vi "CompareRegenModes.vi"() -> ()   [LabVIEW 2014]
doc: "I. Description:\nThis example demonstrates how to continuously output a waveform using an internal sample clock. The automatic regeneration of data has been disabled, so new data has to be provided throughout the duration of the continuous Analog Output operation. This allows the generation of any arbitrary frequency as this VI computes new data for each iteration of the loop, maintaining phase continuity of the signal. The regeneration of data has also been adjusted so that the newest data is output as quickly as possible; thus reducing the lag between the changing of the data and the output of that data.\n\nII. Instructions for Running:\n1. Select the Physical Channel to correspond to where your signal is output on the DAQ device.\n2. Enter the Minimum and Maximum Voltage range.\n3. Specify the desired Sample Clock Rate of the output Waveform. Higher sample clock rates will produce a smoother waveform.\n4. Manually specify the Analog Output buffer size, in number of samples. A larger buffer would help non-regenerative operations avoid errors due to occasional high CPU load. \nNote: \nThe Analog Output buffer has to be at least as big as the amount of data being written to the board per iteration. The recommended buffer size would be at least twice the amount of data being written to the board per iteration.\n5. Enter the Waveform Information. See the documentation of the Basic Function Generator SubVI for information on each parameter.\n\nIII. Block Diagram Steps:\n1. Create an Analog Output Voltage channel.\n2. Configure the task to prohibit the automatic regeneration of data.\n2a. Set the transfer condition to Less than Full. Allows for more rapid updates of Output Buffer.\n3. Call the DAQmx (Sample Clock) VI to set the sample clock rate. Additionally, set the sample mode to Continuous.\n4. Read the actual sample clock rate (eventually coerced depending on the hardware used). \n5. Compute the desired waveform, using the buffer size and the actual update rate. This VI keeps track of the phase of the waveform to ensure that the generated signal is continuous.\n6. Write the waveform to the output buffer. \n7a. Call the Start VI. This is only needed when the loop is executed for the first time.\n7b. Do nothing.\n8. Loop continuously until user presses the Stop button. Every iteration computes and writes a new waveform to the buffer.\n9. Call the Clear Task VI to clear the Task.\n10. Use the popup dialog box to display an error or warning if any.\n\nIV. I/O Connections Overview:\nMake sure your signal output terminal matches the Physical Channel I/O Control. For further connection information, refer to your hardware reference manual."
uses:
  <vilib>/Utility/error.llb/DialogType.ctl
  <vilib>/DAQmx/create/channels.llb/DAQmx Create Virtual Channel.vi
  <vilib>/DAQmx/configure/timing.llb/DAQmx Timing.vi
  <vilib>/DAQmx/write.llb/DAQmx Write.vi
  <vilib>/measure/NI_MABase.lvlib
  <resource>/objmgr/daqmx.rc
panel:
  in  "Regeneration Mode":i32(ring)=10158 items=["Allow Regeneration"=10097, "Do Not Allow Regeneration"=10158]
  in  "Update Buffer":bool
  in  "Stupid Pause":bool
  in  "Size (Samples)":u32=5000
  out "Actual Sample Clock Rate":dbl=20000.0 format="%.2f"
  in  "Sample Clock Rate":dbl=20000.0 format="%0.2f"
  in  "Waveform Type":T1(ring)
  in  "Frequency":dbl=997.0 format="%.2f"
  in  "Amplitude":dbl=1.0 format="%0.2p"
  out "Waveform Graph":waveform(dbl)(graph)={"t0"=timestamp(12.75 s since 1904-01-01), "dt"=5e-05, "Y"=[]} caption="Output Waveform"
  in  "Physical Channels":tag="Dev1/ao0"
  in  "Minimum Value":dbl=-10.0 format="%0.2f"
  in  "Maximum Value":dbl=10.0 format="%0.2f"
  in  "stop":bool
  # "For instructions, select Help>>Show Context Help"
  # "Channel Parameters"
  # "Timing Parameters"
  # "Buffer Parameters"
  # "Waveform Information"
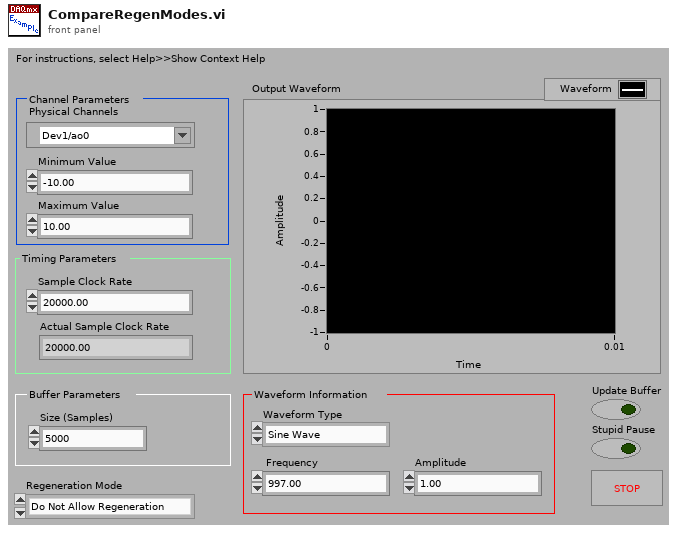
[diagram p1: front panel]
types:
  T1 = enum16{"Sine Wave", "Triangle Wave", "Square Wave", "Sawtooth Wave"}
  T2 = typedef "DialogType.ctl" = u16
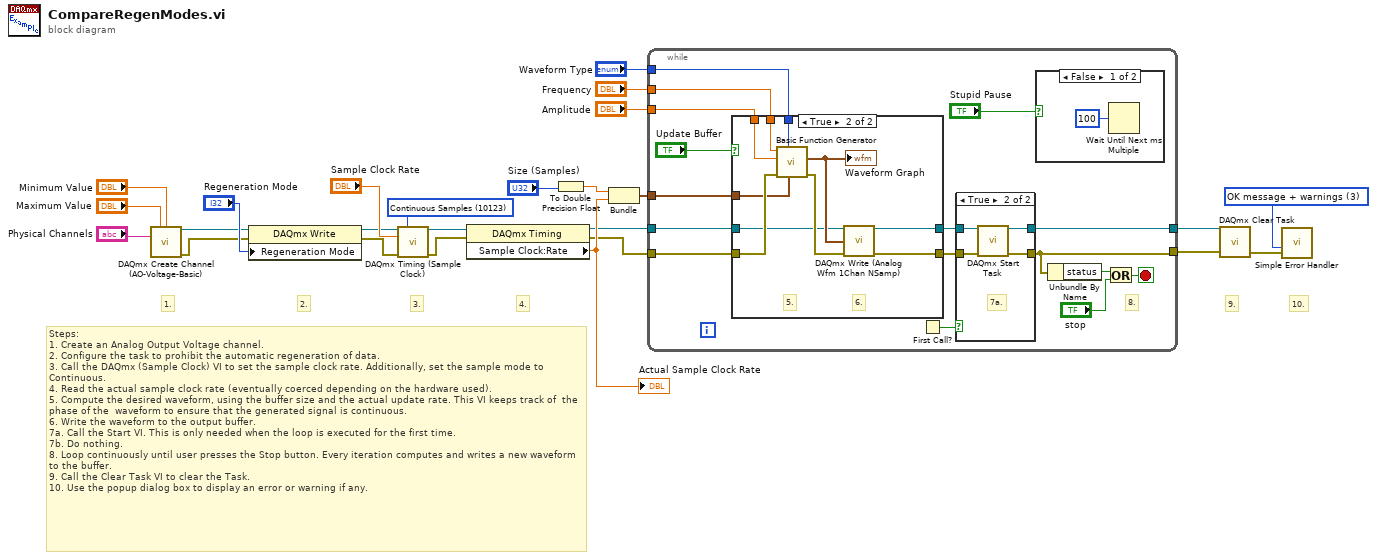
[diagram p0: block diagram]
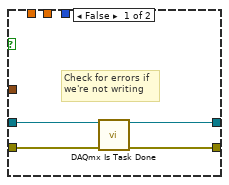
[diagram p2: hidden frame]
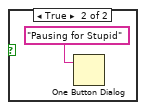
[diagram p3: hidden frame]
diagram:
  w20 = T2 3 items=["no dialog", "OK message", "continue or stop message", "OK message + warnings", "continue/stop + warnings"] ("type of dialog (OK msg:1)")
  w24 = 10123 items=["Finite Samples"=10178, "Continuous Samples"=10123] ("sample mode")
  # "4."
  # "3."
  # "Steps:\n1. Create an Analog Output Voltage channel.\n2. Configure the task to prohibit the automatic regeneration of data. \n3. Call the DAQmx (Sample Clock) VI to set the sample clock rate. Additionally, set the sample mode to Continuous.\n4. Read the actual sample clock rate (eventually coerced depending on the hardware used).\n5. Compute the desired waveform, using the buffer size and the actual update rate. This VI keeps track of  the phase of the  waveform to ensure that the generated signal is continuous.\n6. Write the waveform to the output buffer. \n7a. Call the Start VI. This is only needed when the loop is executed for the first time.\n7b. Do nothing.\n8. Loop continuously until user presses the Stop button. Every iteration computes and writes a new waveform to the buffer.\n9. Call the Clear Task VI to clear the Task.\n10. Use the popup dialog box to display an error or warning if any."
  # "10."
  # "9."
  # "2."
  # "1."
  n1 = call-poly <vilib>:"DAQmx Create Channel (AO-Voltage-Basic).vi"("maximum value"="Maximum Value", "minimum value"="Minimum Value", "physical channels"="Physical Channels") -> ("task out"=w9:refnum<k21>, "error out"=w8:errorcluster)  [unwired: 11 in]
  n2 = property class="DAQmx Write"(reference=w9, error in=w8, "Regeneration Mode"="Regeneration Mode") -> (reference out=w2:refnum<k21>, error out=w1:errorcluster)
  n3 = call-poly <vilib>:"DAQmx Timing (Sample Clock).vi"("task/channels in"=w2, "sample mode"=w24, "rate"="Sample Clock Rate", "error in"=w1) -> ("task out"=w16:refnum<k21>, "error out"=w15:errorcluster)  [unwired: 10 in]
  n4 = property class="DAQmx Timing"(reference=w16, error in=w15) -> (reference out=w6:refnum<k21>, error out=w5:errorcluster, "Sample Clock:Rate"=w14:dbl)
  "Actual Sample Clock Rate" <- w14
  n5 = To Double Precision Float(number="Size (Samples)") -> (double precision float=w3:dbl)
  n6 = Bundle(w3, "SampClk.Rate"=w14) -> (w11:cluster{dbl, "SampClk.Rate":dbl})  [unwired: 1 in]
  n7 = while {
    tunnel: w6 -> [w33]
    tunnel: [w29] -> w19
    tunnel: w5 -> [w38]
    tunnel: [w30] -> w18
    tunnel: "Waveform Type" -> [w37]
    tunnel: "Frequency" -> [w36]
    tunnel: "Amplitude" -> [w35]
    tunnel: w11 -> [w34]
    stop <- w41 stop-if-true
    # "8."
    n8 = case shown="True" "Update Buffer" {
      tunnel: w38 -> [w43 w55]
      tunnel: w37 -> [_ w53]
      tunnel: w36 -> [_ w52]
      tunnel: w35 -> [_ w51]
      tunnel: w34 -> [_ w50]
      tunnel: w33 -> [w45 w48]
      tunnel: [w44 w47] -> w32
      tunnel: [w42 w46] -> w31
      frame False {
        # "Check for errors if\nwe're not writing"
        n9 = call <vilib>:"DAQmx Is Task Done.vi"("task/channels in"=w45, "error in"=w43) -> ("task out"=w44:refnum<k21>, "error out"=w42:errorcluster)  [unwired: 11 in, 1 out]
      }
      frame True {
        # "6."
        # "5."
        n10 = call <vilib>:"Basic Function Generator.vi"("sampling info"=w50, "signal type"=w53, "error in (no error)"=w55, "amplitude"=w51, "frequency"=w52) -> ("error out"=w54:errorcluster, "signal out"=w49:waveform(dbl))  [unwired: 4 in, 1 out]
        "Waveform Graph" <- w49
        n11 = call-poly <vilib>:"DAQmx Write (Analog Wfm 1Chan NSamp).vi"("task/channels in"=w48, "data"=w49, "error in"=w54) -> ("task out"=w47:refnum<k21>, "error out"=w46:errorcluster)  [unwired: 10 in, 1 out]
      }
    }
    n12 = First Call?() -> (First Call?: T/F=w28:bool)
    n13 = case shown="True" w28 {
      tunnel: w32 -> [w59 w63]
      tunnel: w31 -> [w58 w62]
      tunnel: [w58 w61] -> w30
      tunnel: [w59 w60] -> w29
      frame False {
        # "7b."
      }
      frame True {
        # "7a."
        n14 = call <vilib>:"DAQmx Start Task.vi"("task/channels in"=w63, "error in"=w62) -> ("task out"=w60:refnum<k21>, "error out"=w61:errorcluster)  [unwired: 12 in]
      }
    }
    n15 = case shown="False" "Stupid Pause" {
      frame False {
        n16 = Wait Until Next ms Multiple(millisecond multiple=u32 100) -> ()  [unwired: 1 out]
      }
      frame True {
        n17 = One Button Dialog(message="Pausing for Stupid") -> ()  [unwired: 1 in, 1 out]
      }
    }
    n18 = Unbundle By Name(w30) -> ("status"=w40:bool)
    n19 = Or(x=w40, y="stop") -> (x .or. y?=w41:bool)
  }
  n20 = call <vilib>:"DAQmx Clear Task.vi"("task in"=w19, "error in"=w18) -> ("error out"=w25:errorcluster)  [unwired: 13 in]
  n21 = call <vilib>:"Simple Error Handler.vi"("type of dialog (OK msg:1)"=w20, "error in (no error)"=w25) -> ()  [unwired: 3 in, 5 out]
